vi "Set Color Balance.vi"(8 "error in (no error)":errorcluster, 9 "NewVal":T2 {"Blue Gain" min=0 max=10 step=0.05 scale=0.0..10.0 scale format="%#_3g"; "Green Gain" min=0 max=10 step=0.05 scale=0.0..10.0 scale format="%#_3g"; "Red Gain" min=0 max=10 step=0.05 scale=0.0..10.0 scale format="%#_3g"}, 10 "Color Processor References":T1, 11 "TLCamera reference":refnum<k24>) -> (0 "error out":errorcluster, 3 "TLCamera reference out":refnum<k24>)   [LabVIEW 2015]
uses:
  C:/code/Host/Installer/Scientific Camera Interfaces/LabVIEW/32_bit/Library_X86/Thorlabs.TSI.TLCameraInterfaces.dll
  code/Host/Installer/Scientific Camera Interfaces/LabVIEW/32_bit/Library_X86/Thorlabs.TSI.TLCameraInterfaces.dll
  C:/code/Host/Installer/Scientific Camera Interfaces/LabVIEW/32_bit/Library_X86/Thorlabs.TSI.ColorInterfaces.dll
  code/Host/Installer/Scientific Camera Interfaces/LabVIEW/32_bit/Library_X86/Thorlabs.TSI.ColorInterfaces.dll
  Color/Color Processor References.ctl
  Controls/Color Balance.ctl
  C:/code/Host/Installer/Scientific Camera Interfaces/LabVIEW/32_bit/Library_X86/Thorlabs.TSI.ColorProcessor.dll
  code/Host/Installer/Scientific Camera Interfaces/LabVIEW/32_bit/Library_X86/Thorlabs.TSI.ColorProcessor.dll
  C:/code/Host/Installer/Scientific Camera Interfaces/LabVIEW/32_bit/Library_X86/Thorlabs.TSI.Demosaicker.dll
  code/Host/Installer/Scientific Camera Interfaces/LabVIEW/32_bit/Library_X86/Thorlabs.TSI.Demosaicker.dll
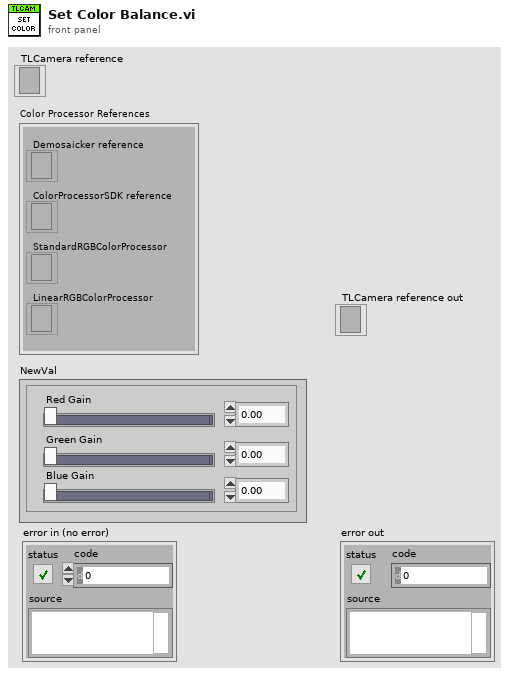
[diagram p1: front panel]
types:
  T1 = typedef "Color Processor References.ctl" = cluster{"Demosaicker reference":refnum<k24>, "ColorProcessorSDK reference":refnum<k24>, "StandardRGBColorProcessor":refnum<k24>, "LinearRGBColorProcessor":refnum<k24>}
  T2 = typedef "Color Balance.ctl" = cluster{"Red Gain":sgl, "Green Gain":sgl, "Blue Gain":sgl}
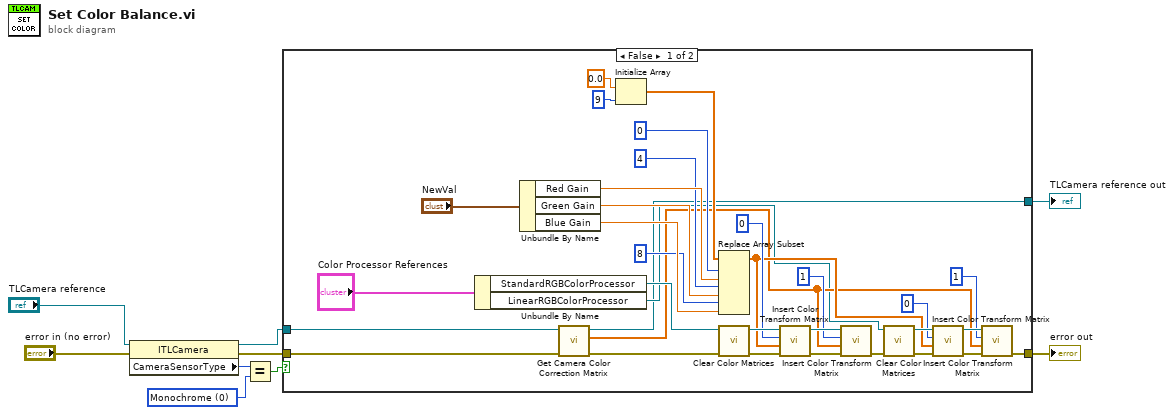
[diagram p0: block diagram]
diagram:
  w4 = 0 items=["Monochrome", "Bayer"] ("CameraSensorType")
  n1 = property class="ITLCamera"(reference="TLCamera reference", error in="error in (no error)") -> (reference out=w3:refnum<k24>, error out=w2:errorcluster, "CameraSensorType"=w5:i32)
  n2 = Equal?(x=w5, y=w4) -> (x = y?=w1:bool)
  n3 = case shown="False" w1 {
    tunnel: [w11 w43] -> w9
    tunnel: [w10 w44] -> w8
    tunnel: w3 -> [w24 w44]
    tunnel: w2 -> [w23 w43]
    frame False {
      n4 = Unbundle By Name("Color Processor References") -> ("StandardRGBColorProcessor"=w31:refnum<k24>, "LinearRGBColorProcessor"=w12:refnum<k24>)
      n5 = Unbundle By Name("NewVal") -> ("Red Gain"=w40:sgl, "Green Gain"=w41:sgl, "Blue Gain"=w42:sgl)
      n6 = call "Get Camera Color Correction Matrix.vi"("error in (no error)"=w23, "TLCamera reference"=w24) -> ("error out"=w22:errorcluster, "Camera Color Correction Matrix"=w13:sgl[], "TLCamera reference out"=w10:refnum<k24>)  [unwired: 7 in]
      n7 = Initialize Array(sgl 0.0 ("element"), 9 ("dimension size")) -> (w37:sgl[])
      n8 = Replace Array Subset(array=w37, new element #1=w40, index #1=0 ("index"), new element #2=w41, index #2=4 ("index"), new element #3=w42, index #3=8 ("index")) -> (w14:sgl[])
      n9 = call "Clear Color Matrices.vi"("error in (no error)"=w22, "ColorProcessor reference in"=w31) -> ("error out"=w28:errorcluster, "ColorProcessor reference out"=w30:refnum<k24>)  [unwired: 8 in]
      n10 = call "Insert Color Transform Matrix.vi"("error in (no error)"=w28, "colorTransformMatrix"=w14, "index"=0, "ColorProcessor reference in"=w30) -> ("error out"=w27:errorcluster, "ColorProcessor reference out"=w26:refnum<k24>)  [unwired: 6 in]
      n11 = call "Insert Color Transform Matrix.vi"("error in (no error)"=w27, "colorTransformMatrix"=w13, "index"=1, "ColorProcessor reference in"=w26) -> ("error out"=w15:errorcluster)  [unwired: 6 in, 1 out]
      n12 = call "Clear Color Matrices.vi"("error in (no error)"=w15, "ColorProcessor reference in"=w12) -> ("error out"=w19:errorcluster, "ColorProcessor reference out"=w21:refnum<k24>)  [unwired: 8 in]
      n13 = call "Insert Color Transform Matrix.vi"("error in (no error)"=w19, "colorTransformMatrix"=w14, "index"=0, "ColorProcessor reference in"=w21) -> ("error out"=w18:errorcluster, "ColorProcessor reference out"=w17:refnum<k24>)  [unwired: 6 in]
      n14 = call "Insert Color Transform Matrix.vi"("error in (no error)"=w18, "colorTransformMatrix"=w13, "index"=1, "ColorProcessor reference in"=w17) -> ("error out"=w11:errorcluster)  [unwired: 6 in, 1 out]
    }
    frame True {
    }
  }
  "TLCamera reference out" <- w8
  "error out" <- w9
